vi "Example Simple.vi"() -> ()   [LabVIEW 2010]
uses:
  C:/tf/play/labview/Tinkerforge.dll
  Tinkerforge.dll
panel:
  out "voltage (V)":sgl
  out "current (A)":sgl
  in  "uid":string="amb"
  in  "port":i32=4223
  in  "host":string="localhost"
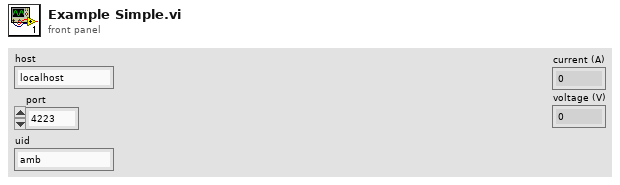
[diagram p1: front panel]
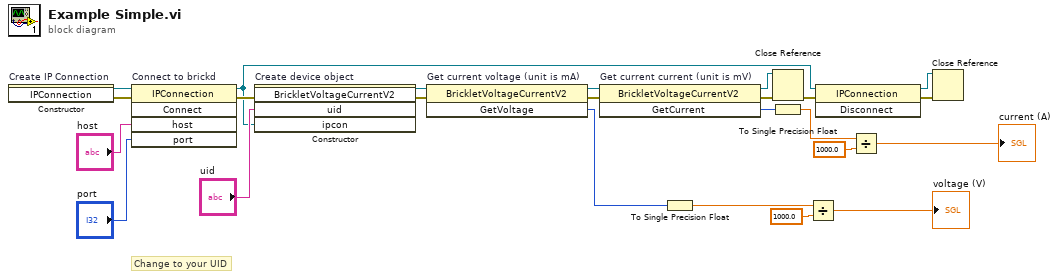
[diagram p0: block diagram]
diagram:
  # "Change to your UID"
  n1 = constructor on="Create IP Connection" class="IPConnection"() -> (reference out=w24:refnum<k24>, error out=w10:errorcluster)  [unwired: 3 in, 1 out]
  n2 = invoke on="Connect to brickd" class="IPConnection" method="Connect"(reference=w24, error in=w10, "host"="host", "port"="port") -> (reference out=w15:refnum<k24>, error out=w20:errorcluster)  [unwired: 1 in, 3 out]
  n3 = constructor on="Create device object" class="BrickletVoltageCurrentV2"(error in=w20, "uid"="uid", "ipcon"=w15) -> (reference out=w18:refnum<k24>, error out=w19:errorcluster)  [unwired: 2 in, 3 out]
  n4 = invoke on="Get current voltage (unit is mA)" class="BrickletVoltageCurrentV2" method="GetVoltage"(reference=w18, error in=w19) -> (reference out=w8:refnum<k24>, error out=w9:errorcluster, "GetVoltage"=w1:i32)  [unwired: 1 in]
  n5 = invoke on="Get current current (unit is mV)" class="BrickletVoltageCurrentV2" method="GetCurrent"(reference=w8, error in=w9) -> (reference out=w6:refnum<k24>, error out=w7:errorcluster, "GetCurrent"=w2:i32)  [unwired: 1 in]
  n6 = To Single Precision Float(number=w1) -> (single precision float=w3:sgl)
  n7 = Close Reference(reference=w6, error in (no error)=w7) -> (error out=w17:errorcluster)
  n8 = To Single Precision Float(number=w2) -> (single precision float=w12:sgl)
  n9 = Divide(x=w3, y=sgl 1000.0) -> (x/y=→"voltage (V)":sgl)
  n10 = invoke class="IPConnection" method="Disconnect"(reference=w15, error in=w17) -> (reference out=w14:refnum<k24>, error out=w16:errorcluster)  [unwired: 1 in, 1 out]
  n11 = Divide(x=w12, y=sgl 1000.0) -> (x/y=→"current (A)":sgl)
  n12 = Close Reference(reference=w14, error in (no error)=w16) -> ()  [unwired: 1 out]
